vi "LJM_IPToNumber.vi"(8 "error in":errorcluster, 10 "IPv4String":string) -> (0 "error out":errorcluster, 2 "Number":u32)   [LabVIEW 2024]
uses:
  labjackm.dll
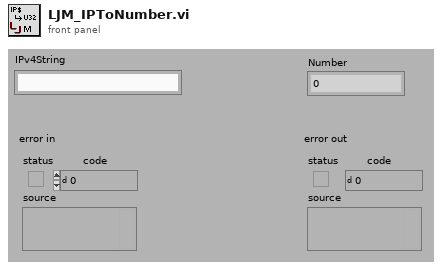
[diagram p1: front panel]
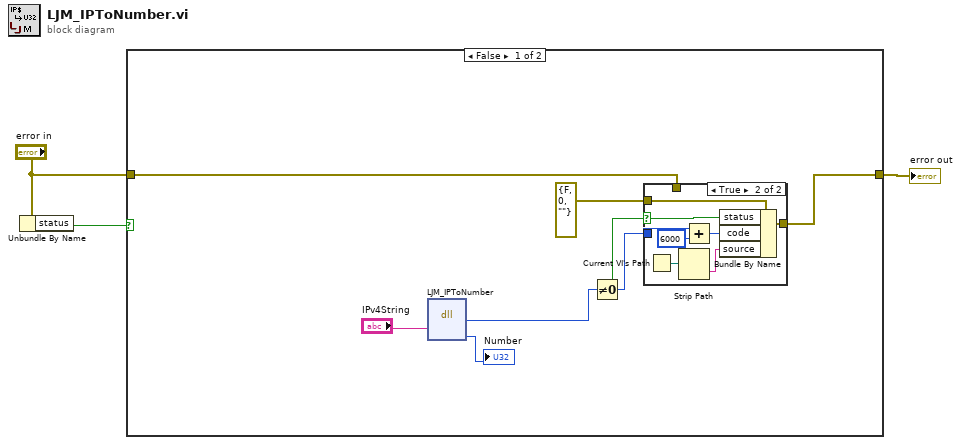
[diagram p0: block diagram]
diagram:
  n1 = Unbundle By Name("error in") -> ("status"=w3:bool)
  n2 = case shown="False" w3 {
    tunnel: "error in" -> [w7 w20]
    tunnel: [w6 w20] -> w1
    frame False {
      n3 = dll-call lib="labjackm.dll" fn="LJM_IPToNumber"("IPv4String"="IPv4String") -> (w10:i32, "Number"=→"Number":u32)  [unwired: 5 in, 2 out]
      n4 = Not Equal To 0?(x=w10) -> (x != 0?=w9:bool)
      n5 = case shown="True" w9 {
        selector: w9 -> [_ w18]
        tunnel: [w11 w19] -> w6
        tunnel: errorcluster {"status"=FALSE, "code"=0, "source"=""} ("error IO") -> [_ w17]
        tunnel: w10 -> [_ w13]
        tunnel: w7 -> [w11 _]
        frame False {
        }
        frame True {
          n6 = Current VI's Path() -> (path=w15:path)
          n7 = Strip Path(path=w15) -> (name=w16:string)  [unwired: 1 out]
          n8 = Add(x=w13, y=6000) -> (x+y=w14:i32)
          n9 = Bundle By Name(cluster=w17, "status"=w18, "code"=w14, "source"=w16) -> (w19:errorcluster)
        }
      }
    }
    frame True {
    }
  }
  "error out" <- w1
